vi "Observe Data.vi"(6 "Time Stamp":timestamp, 8 "error in (no error)":errorcluster, 9 "Value":variant, 10 "Datum Name":string, 11 "MediatorBusMonitor in":refnum<class "MediatorBusMonitor.lvclass">) -> (0 "error out":errorcluster, 3 "MediatorBusMonitor out":refnum<class "MediatorBusMonitor.lvclass">)   [LabVIEW 2015, in "Mediator.lvlib" / "MediatorBusMonitor.lvclass"]
doc: "<License>\nCopyright © 2017 Composed Systems, LLC | All rights reserved\nwww.composed.io\n\nAuthor: Ethan Stern <ethan.stern@composed.io>\n\nThis software is provided \"AS IS\" WITHOUT WARRANTIES, either express or implied, AND IS FOR EDUCATIONAL PURPOSES ONLY.\n</License>"
uses:
  MediatorBusMonitor.lvclass
  MediatorBusMonitor.lvclass/MediatorBusMonitor.ctl
  Components/CurrentValueTable/CurrentValueTable.lvclass
  Components/VariantExtensions/VariantExtensions.lvlib
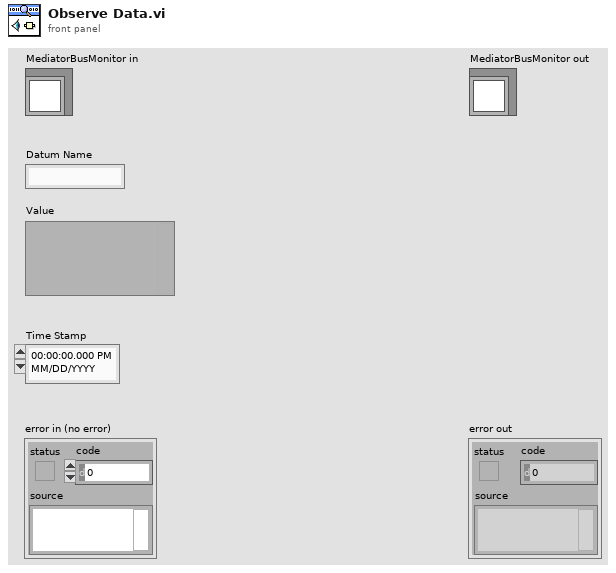
[diagram p1: front panel]
types:
  T1 = typedef "CurrentValueTable.lvlib/CurrentValueTable.lvclass/CurrentValueTable Reference.ctl" = refnum<data-value>
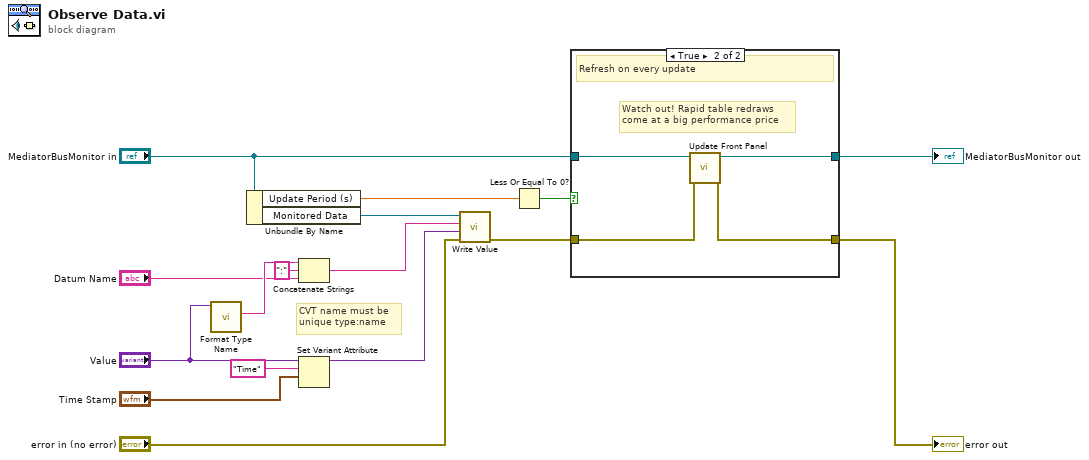
[diagram p0: block diagram]
diagram:
  # "CVT name must be\nunique type:name"
  n1 = call "Format Type Name.vi"("Data Type"="Value") -> ("Type Name"=w4:string)  [unwired: 9 in, 1 out]
  n2 = Unbundle By Name("MediatorBusMonitor in") -> ("Update Period (s)"=w13:dbl, "Monitored Data"=w16:T1)
  n3 = Concatenate Strings(w4, ":" ("string"), "Datum Name") -> (w1:string)
  n4 = Set Variant Attribute(Variant="Value", name="Time", value="Time Stamp") -> (Variant out=w7:variant)  [unwired: 1 in, 2 out]
  n5 = call "Write Value.vi"("error in (no error)"="error in (no error)", "Value"=w7, "Data Name (Use Value Name)"=w1, "Current Value Table"=w16) -> ("error out"=w11:errorcluster)  [unwired: 6 in, 1 out]
  n6 = Less Or Equal To 0?(x=w13) -> (x <= 0?=w9:bool)
  n7 = case shown="True" w9 {
    tunnel: "MediatorBusMonitor in" -> [w17 w22]
    tunnel: [w17 w21] -> w12
    tunnel: w11 -> [w18 w20]
    tunnel: [w18 w19] -> w10
    frame False {
      # "Timed message triggers updates"
    }
    frame True {
      # "Watch out! Rapid table redraws\ncome at a big performance price"
      # "Refresh on every update"
      n8 = call "Update Front Panel.vi"("error in (no error)"=w20, "MediatorBusMonitor In"=w22) -> ("error out"=w19:errorcluster, "MediatorBusMonitor Out"=w21:refnum<class "MediatorBusMonitor.lvclass">)  [unwired: 8 in]
    }
  }
  "error out" <- w10
  "MediatorBusMonitor out" <- w12
